vi "Lookup Group.vi"(7 "Group Type (Abstract)":refnum<class "GroupAbstract.lvclass">, 8 "error in (no error)":errorcluster, 10 "Group Name":string, 11 "ChannelService in":refnum<class "ChannelService.lvclass">) -> (0 "error out":errorcluster, 2 "Group":refnum<class "GroupAbstract.lvclass">, 3 "ChannelService out":refnum<class "ChannelService.lvclass">)   [LabVIEW 2020, in "Vecto.lvlib" / "ChannelService.lvclass"]
uses:
  ChannelService.lvclass
  GroupAbstract/GroupAbstract.lvclass
  GroupValue/GroupAbstractValue.lvclass
  C:/dev/lv20CE/relink/lv-promises/Promises/Value/Value.lvclass
  Lookup Group Data.ctl
  Lookup Type.ctl
  lv-promises/Promises/Promise/Promise.lvclass
  ChannelService.lvclass/ChannelService.ctl
  lv-promises/Promises/Promise/Promise.lvclass/Promise.ctl
  lv-promises/Promises/Future/Future.lvclass/Future.ctl
  GroupValue/GroupAbstractValue.lvclass/GroupAbstractValue.ctl
  lv-promises/Promises/Future/Future.lvclass
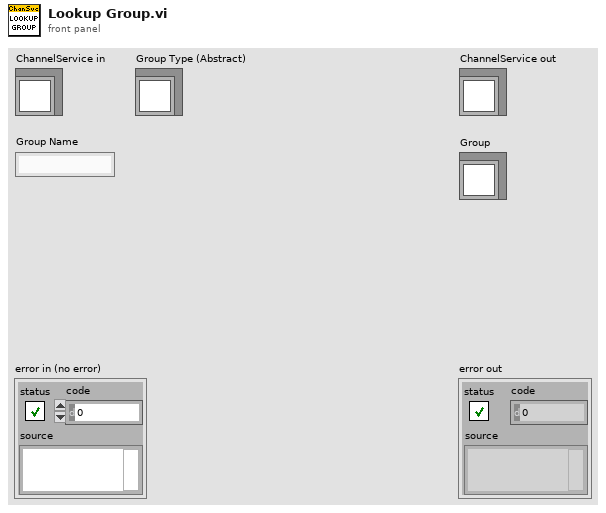
[diagram p1: front panel]
types:
  T1 = typedef "Vecto.lvlib/ChannelService.lvclass/Lookup Type.ctl" = enum16{"Name", "Node", "Pattern"}
  T2 = typedef "Vecto.lvlib/ChannelService.lvclass/Lookup Group Data.ctl" = cluster{"Type":T1, "Group Lookup":string, "Node Lookup":string, "Promise":refnum<class "Promise.lvclass">}
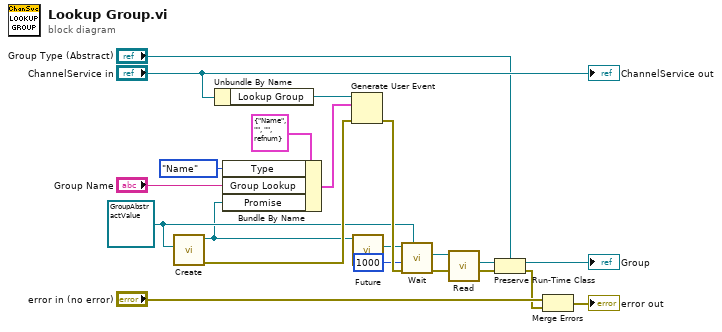
[diagram p0: block diagram]
diagram:
  w16 = refnum<class "GroupAbstractValue.lvclass"> refnum ("Vecto.lvlib:GroupValue.lvclass")
  n1 = call "Create.vi"("Result Type"=w16) -> ("error out"=w19:errorcluster, "Promise"=w9:refnum<class "Promise.lvclass">)  [unwired: 9 in]
  n2 = Unbundle By Name("ChannelService in") -> ("Lookup Group"=w12:refnum<user-event>)
  n3 = Bundle By Name(cluster=T2 {"Type"=enum."Name", "Group Lookup"="", "Node Lookup"="", "Promise"=refnum} ("event data"), "Type"=Lookup_Type."Name" ("Lookup Type"), "Group Lookup"="Group Name", "Promise"=w9) -> (w8:T2)
  n4 = Generate User Event(user event=w12, event data cluster=w8, error in=w19) -> (error out=w20:errorcluster)  [unwired: 1 in, 1 out]
  n5 = call "Future.vi"("Promise in"=w9) -> ("Future"=w17:refnum<class "Future.lvclass">)  [unwired: 9 in, 1 out]
  n6 = call "Wait.vi"("Result Type"=w16, "error in (no error)"=w20, "Timeout mS (-1)"=1000, "Future in"=w17) -> ("error out"=w4:errorcluster, "Result"=w14:refnum<class "GroupAbstractValue.lvclass">)  [unwired: 6 in]
  n7 = call "Read.vi"("GroupValue in"=w14) -> ("Group"=w7:refnum<class "GroupAbstract.lvclass">)  [unwired: 10 in]
  n8 = Preserve Run-Time Class(object in=w7, error in=w4, 2:"Group Type (Abstract)") -> (object out=→"Group":refnum<class "GroupAbstract.lvclass">, error out=w3:errorcluster)
  n9 = Merge Errors("error in (no error)", w3) -> (→"error out":errorcluster)
  "ChannelService out" <- "ChannelService in"
